vi "setChannelStatus.vi"(7 "Chn":string, 8 "error in (no error)":errorcluster, 10 "State":bool, 11 "ScopeNi in":refnum<class "ScopeNi.lvclass">) -> (0 "error out":errorcluster, 3 "ScopeNi out":refnum<class "ScopeNi.lvclass">)   [LabVIEW 2023, in "ScopeNi.lvclass"]
doc: "<b>Author:</b> Wolfgang\n<b>Description:</b> Enable/Disable a Channel from being visible."
uses:
  ScopeNi.lvclass
  ScopeNi.lvclass/ScopeNi.ctl
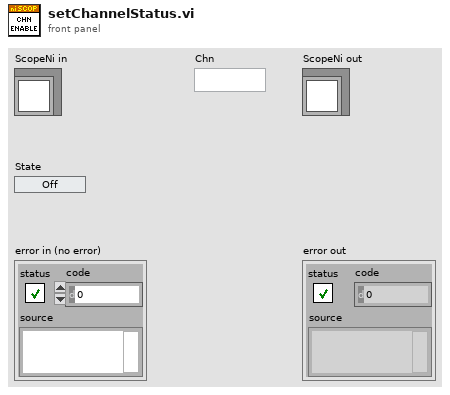
[diagram p1: front panel]
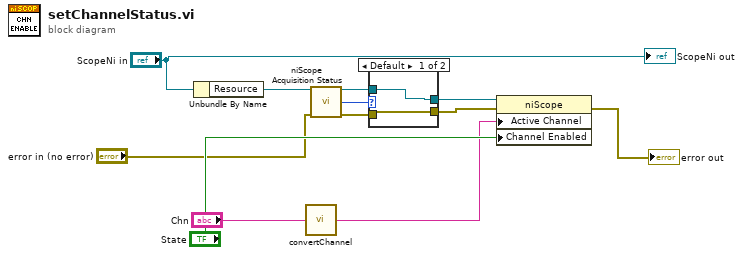
[diagram p0: block diagram]
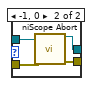
[diagram p2: hidden frame]
diagram:
  n1 = Unbundle By Name("ScopeNi in") -> ("Resource"=w7:refnum<k15>)
  n2 = call "convertChannel.vi"("Chn in"="Chn") -> ("Chn out"=w8:string)
  n3 = call <instrlib>:"niScope Acquisition Status.vi"("instrument handle"=w7, "error in"="error in (no error)") -> ("instrument handle out"=w5:refnum<k15>, "acquisition status"=w6:i32, "error out"=w1:errorcluster)  [unwired: 11 in]
  n4 = case shown="Default" w6 {
    tunnel: w5 -> [w14 w18]
    tunnel: [w14 w17] -> w3
    tunnel: [w13 w16] -> w2
    tunnel: w1 -> [w13 w15]
    frame Default {
    }
    frame -1, 0 {
      n5 = call <instrlib>:"niScope Abort.vi"("instrument handle"=w18, "error in"=w15) -> ("instrument handle out"=w17:refnum<k15>, "error out"=w16:errorcluster)  [unwired: 12 in]
    }
  }
  n6 = property class="niScope"(reference=w3, error in=w2, "Active Channel"=w8, "Channel Enabled"="State") -> (error out=→"error out":errorcluster)  [unwired: 1 out]
  "ScopeNi out" <- "ScopeNi in"
